vi "ERR HANDLER - Demo.vi"() -> ()   [LabVIEW 2013]
panel:
  out "Last Error":errorcluster
  out "Error Count":i32
  in  "Inject":bool
  in  "Error":errorcluster={"status"=TRUE, "code"=7, "source"="here.vi"}
  in  "Stop":bool
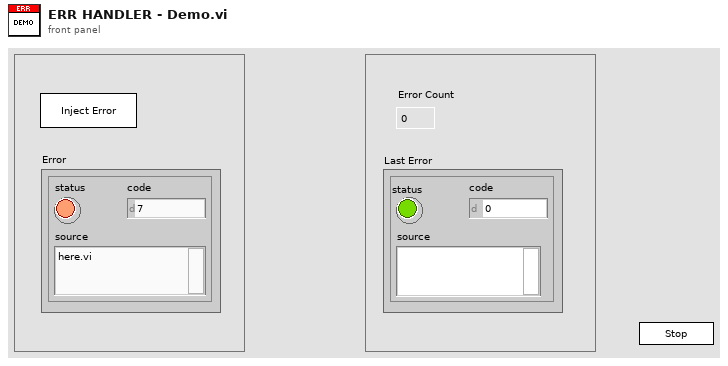
[diagram p1: front panel]
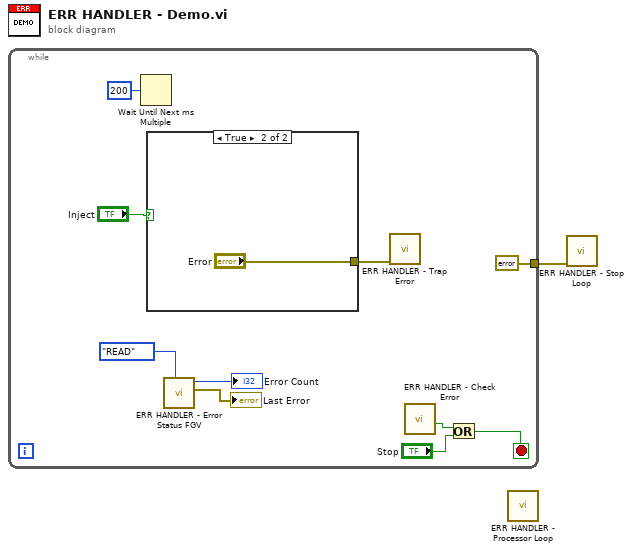
[diagram p0: block diagram]
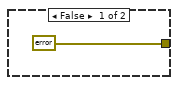
[diagram p2: hidden frame]
diagram:
  n1 = while {
    tunnel: [errorcluster {"status"=FALSE, "code"=0, "source"=""} ("error in")] -> w1
    stop <- w9 stop-if-true
    n2 = Wait Until Next ms Multiple(millisecond multiple=u32 200) -> ()  [unwired: 1 out]
    n3 = case shown="True" "Inject" {
      tunnel: [errorcluster {"status"=FALSE, "code"=0, "source"=""} ("Error In") "Error"] -> w6
      frame False {
      }
      frame True {
      }
    }
    n4 = call "ERR HANDLER - Error Status FGV.vi"("Method"=enum16{"READ", "WRITE"}."READ") -> ("Last Error (R)"=→"Last Error":errorcluster, "Error Count (R)"=→"Error Count":i32)  [unwired: 8 in, 1 out]
    n5 = call "ERR HANDLER - Trap Error.vi"("error in"=w6) -> ()  [unwired: 11 in]
    n6 = call "ERR HANDLER - Check Error.vi"() -> ("ABORT"=w10:bool)  [unwired: 11 in]
    n7 = Or(x=w10, y="Stop") -> (x .or. y?=w9:bool)
  }
  n8 = call "ERR HANDLER - Processor Loop.vi"() -> ()  [unwired: 12 in]
  n9 = call "ERR HANDLER - Stop Loop.vi"("error in"=w1) -> ()  [unwired: 10 in, 1 out]
